vi "ParseOutDataAndRegisterType.vi"(11 "DataType(:RegisterType) in":string) -> (2 "RegisterType":string, 3 "DataType":string)   [LabVIEW 2018]
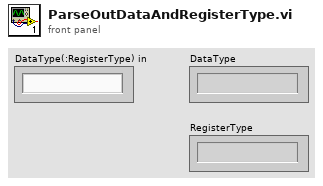
[diagram p1: front panel]
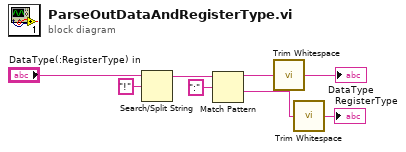
[diagram p0: block diagram]
diagram:
  n1 = Search/Split String(string="DataType(:RegisterType) in", search string/char (-)="!") -> (substring before match=w6:string)  [unwired: 1 in, 2 out]
  n2 = Match Pattern(string=w6, regular expression=":") -> (before substring=w4:string, after substring=w5:string)  [unwired: 1 in, 2 out]
  n3 = call <vilib>:"Trim Whitespace.vi"("string"=w4) -> ("trimmed string"=→"DataType":string)  [unwired: 1 in]
  n4 = call <vilib>:"Trim Whitespace.vi"("string"=w5) -> ("trimmed string"=→"RegisterType":string)  [unwired: 1 in]
